vi "teststreamer nowait server.vi"() -> ()   [LabVIEW 2016]
uses:
  dllwrapper/action complete event.ctl
  tls classes/connection creator/server acceptor/server acceptor.lvclass
  C:/Users/IEUser/Desktop/libasynclvtls/tls classes/connection creator/connection creator.lvclass
  tls classes/engine context/engine context.lvclass
  tls classes/connection/connection.lvclass
  tls classes/connection creator/connection creator.lvclass
  dllwrapper/async tls dl.lvlib
  <vilib>/ptbypt/NI_PtbyPt.lvlib
panel:
  in  "dimension size":i32=20000
  in  "Numeric 2":i32=1
  in  "thread count":u64=2
  out "Numeric":dbl
  out "Waveform Chart":dbl(graph)
  out "bytes/s":dbl format="%^#_9e"
  out "bytes written":i32
  in  "stop":bool
  out "error out 3":errorcluster
  out "error out 2":errorcluster
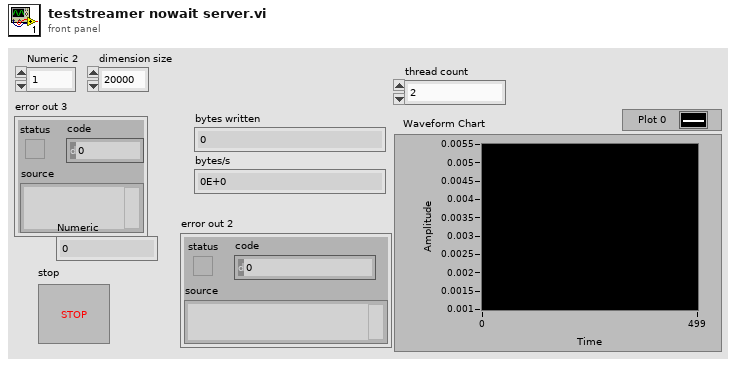
[diagram p1: front panel]
types:
  T1 = typedef "async tls dl.lvlib/action complete event.ctl" = cluster{"request ID":u32, "error code":i32, "error string":string}
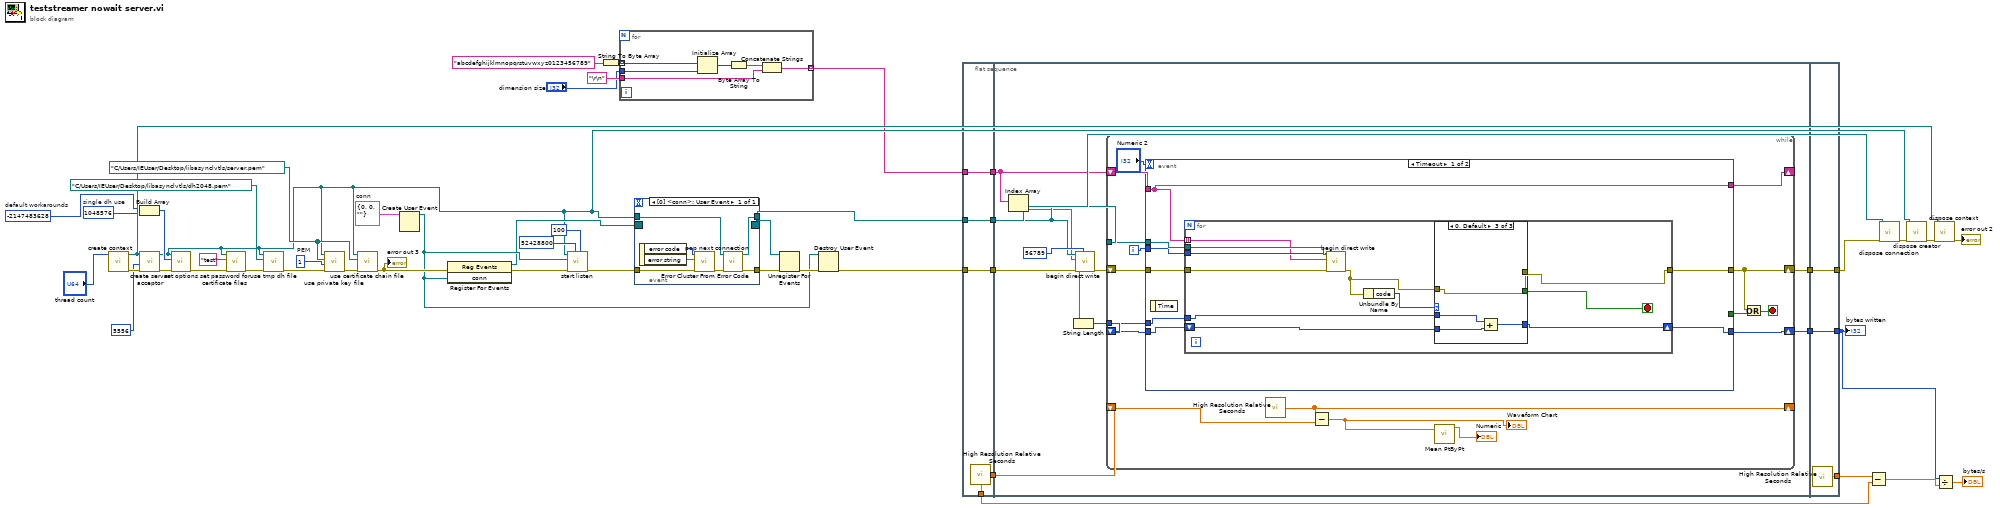
[diagram p0: block diagram]
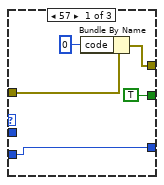
[diagram p2: hidden frame]
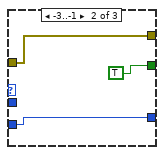
[diagram p3: hidden frame]
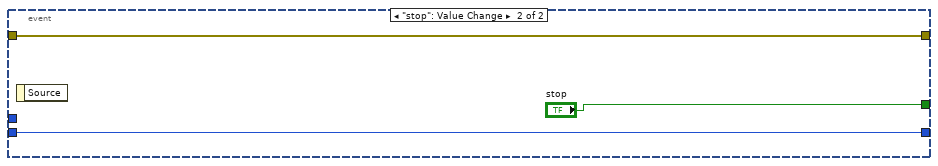
[diagram p4: hidden frame]
diagram:
  w30 = T1 {"request ID"=0, "error code"=0, "error string"=""}  # conn
  w35 = 1  # PEM
  w40 = path "C:/Users/IEUser/Desktop/libasynclvtls/server.pem" ("cert chain file")
  w43 = -2147483628  # default workarounds
  w44 = 1048576  # single dh use
  n1 = call "create context.vi"("thread count"="thread count") -> ("error out"=w47:errorcluster, "engine context out"=w46:refnum<class "engine context.lvclass">)  [unwired: 9 in]
  n2 = Build Array(w43, w44) -> (w37:i32[])
  n3 = call "create server acceptor.vi"("error in"=w47, "port"=u16 5556, "engine context in"=w46) -> ("error out"=w45:errorcluster, "server acceptor out"=w20:refnum<class "server acceptor.lvclass">)  [unwired: 7 in]
  n4 = call "set options.vi"("error in"=w45, "options"=w37, "connection creator in"=w20) -> ("error out"=w42:errorcluster)  [unwired: 8 in]
  n5 = call "set password for certificate files.vi"("error in"=w42, "password"="test" ("file"), "connection creator in"=w20) -> ("error out"=w34:errorcluster)  [unwired: 8 in]
  n6 = call "use tmp dh file.vi"("error in"=w34, "tmp dh file"=path "C:/Users/IEUser/Desktop/libasynclvtls/dh2048.pem", "connection creator in"=w20) -> ("error out"=w33:errorcluster)  [unwired: 8 in]
  n7 = call "use private key file.vi"("error in"=w33, "format"=w35, "private key file"=w40, "connection creator in"=w20) -> ("error out"=w32:errorcluster)  [unwired: 7 in]
  n8 = call "use certificate chain file.vi"("error in"=w32, "cert chain file"=w40, "connection creator in"=w20) -> ("error out"=w39:errorcluster)  [unwired: 8 in]
  "error out 3" <- w39
  n9 = Create User Event(user event datatype=w30) -> (user event=w26:refnum<user-event>)  [unwired: 1 in, 1 out]
  n10 = register-events(error in=w39, w26) -> (reference out=w22:refnum<event-registration>, error out=w29:errorcluster)  [unwired: 1 in]
  n11 = call "start listen.vi"("output chunk queue size"=u64 100, "stream buffer size"=u64 52428800, "error in"=w29, "completion event"=w26, "server acceptor in"=w20) -> ("error out"=w24:errorcluster)  [unwired: 6 in]
  n12 = String To Byte Array(string="abcdefghijklmnopqrstuvwxyz0123456789") -> (unsigned byte array=w18:u8[])
  n13 = for {
    tunnel: w18 -> [w56] mode=indexing
    tunnel: [w53] -> w3 mode=indexing
    tunnel: "\r\n" ("termination") -> [w52]
    tunnel: "dimension size" -> [w51]
    n14 = Initialize Array(w56, w51) -> (w55:u8[])
    n15 = Byte Array To String(unsigned byte array=w55) -> (string=w54:string)
    n16 = Concatenate Strings(w54, w52) -> (w53:string)
  }
  n17 = event shown="[0] <conn>: User Event" {
    selector: w22 -> [_]
    dyn-events: [_] -> w23
    timeout: _ -> [_]
    tunnel: [w62] -> w25
    tunnel: w24 -> [w63]
    tunnel: w20 -> [w58]
    tunnel: [w57] -> w19
    event User Event {
      n18 = event-data() -> ("error code"=w60:i32, "error string"=w59:string)  [unwired: 1 in]
      n19 = call <vilib>:"Error Cluster From Error Code.vi"("error in (no error)"=w63, "error message (\"\")"=w59, "error code (0)"=w60) -> ("error out"=w61:errorcluster)  [unwired: 6 in]
      n20 = call "pop next connection.vi"("error in"=w61, "connection creator in"=w58) -> ("error out"=w62:errorcluster, "connection out"=w57:refnum<class "connection.lvclass">)  [unwired: 8 in]
    }
  }
  n21 = Unregister For Events(event registration refnum=w23, error in=w25) -> (error out=w28:errorcluster)
  n22 = Destroy User Event(user event=w26, error in=w28) -> (error out=w27:errorcluster)
  n23 = flat-sequence {
    tunnel: w3 -> [w65]
    tunnel: w19 -> [w66]
    tunnel: w27 -> [w67]
    tunnel: [w67] -> w15
    tunnel: [w66] -> w14
    tunnel: [w65] -> w13
    tunnel: [w64] -> w10
    tunnel: [w64] -> w4
    tunnel: w15 -> [w75]
    tunnel: w14 -> [w73]
    tunnel: w13 -> [w72]
    tunnel: [w74] -> w12
    tunnel: [w69] -> w9
    tunnel: w4 -> [w68]
    tunnel: [w130] -> w21
    tunnel: w12 -> [w130]
    tunnel: [w129] -> w11
    tunnel: [w128] -> w7
    tunnel: w9 -> [w128]
    frame #0 {
      n24 = call <vilib>:"High Resolution Relative Seconds.vi"() -> ("relative seconds"=w64:dbl)
    }
    frame #1 {
      n25 = Index Array(array=w72) -> (element=w71:string)  [unwired: 1 in]
      n26 = String Length(string=w71) -> (length=w70:i32)
      n27 = call "begin direct write.vi"("id"=u32 56789, "error in"=w75, "data"=w71, "connection in"=w73) -> ("error out"=w76:errorcluster)  [unwired: 6 in, 1 out]
      n28 = while {
        shift-right: [w90] -> w74
        shift-left: w76 -> [w93]
        tunnel: w73 -> [w92]
        shift-right: [w87] -> _
        shift-left: w72 -> [w88]
        tunnel: w70 -> [w85]
        shift-right: [w84] -> w69
        shift-left: w70 -> [w83]
        shift-right: [w81] -> _
        shift-left: w68 -> [w82]
        i -> [w86]
        stop <- w91 stop-if-true
        n29 = event shown="[0] Timeout" {
          selector: _ -> [_ _]
          dyn-events: _ -> [_ _]
          timeout: "Numeric 2" -> [_ _]
          tunnel: w93 -> [w101 w126]
          tunnel: w92 -> [w99 _]
          tunnel: [w100 w126] -> w90
          tunnel: [_ "stop"] -> w89
          tunnel: w88 -> [w94 _]
          tunnel: [w94 _] -> w87
          tunnel: w86 -> [w98 _]
          tunnel: w85 -> [w95 _]
          tunnel: [w97 w125] -> w84
          tunnel: w83 -> [w96 w125]
          event Timeout {
            n30 = event-data() -> ()  [unwired: 1 in, 1 out]
            n31 = for {
              tunnel: w99 -> [w111]
              tunnel: w98 -> [w110]
              tunnel: w95 -> [w107]
              shift-right: [w109] -> w97
              shift-left: w96 -> [w108]
              tunnel: w94 -> [w106] mode=indexing
              tunnel: w101 -> [w112]
              tunnel: [w103] -> w100
              stop <- w104 stop-if-true
              n32 = call "begin direct write.vi"("id"=w110, "error in"=w112, "data"=w106, "connection in"=w111) -> ("error out"=w102:errorcluster)  [unwired: 6 in, 1 out]
              n33 = Unbundle By Name(w102) -> ("code"=w105:i32)
              n34 = case shown="0, Default" w105 {
                tunnel: [w117 w120 w124] -> w109
                tunnel: w108 -> [w117 w120 w123]
                tunnel: w107 -> [_ _ w122]
                tunnel: [TRUE TRUE _] -> w104
                tunnel: [w115 w118 w121] -> w103
                tunnel: w102 -> [w116 w118 w121]
                frame 57 {
                  n35 = Bundle By Name(cluster=w116, "code"=0) -> (w115:errorcluster)
                }
                frame -3..-1 {
                }
                frame 0, Default {
                  n36 = Add(x=w122, y=w123) -> (x+y=w124:i32)
                }
              }
            }
          }
          event "stop": Value Change {
            n37 = event-data() -> ()  [unwired: 1 in, 1 out]
          }
        }
        n38 = call <vilib>:"High Resolution Relative Seconds.vi"() -> ("relative seconds"=w81:dbl)
        n39 = Subtract(x=w81, y=w82) -> (x-y=w79:dbl)
        "Waveform Chart" <- w79
        n40 = call <vilib>:"Mean PtByPt.vi"("x"=w79) -> ("mean"=→"Numeric":dbl)  [unwired: 3 in, 1 out]
        n41 = Or(x=w90, y=w89) -> (x .or. y?=w91:bool)
      }
    }
    frame #2 {
      n42 = call <vilib>:"High Resolution Relative Seconds.vi"() -> ("relative seconds"=w129:dbl)
    }
  }
  n43 = Subtract(x=w11, y=w10) -> (x-y=w8:dbl)
  n44 = call "dispose connection.vi"("error in"=w21, "connection in"=w19) -> ("error out"=w50:errorcluster)  [unwired: 9 in]
  n45 = call "dispose creator.vi"("error in"=w50, "connection creator in"=w20) -> ("error out"=w49:errorcluster)  [unwired: 9 in]
  n46 = call "dispose context.vi"("error in"=w49, "engine context out"=w46) -> ("error out"=→"error out 2":errorcluster)  [unwired: 9 in]
  n47 = Divide(x=w7, y=w8) -> (x/y=→"bytes/s":dbl)
  "bytes written" <- w7
